vi "e.gate HighSpeedPort Decode Diagnostic Data.vi"(8 "error in":errorcluster, 10 "IsBigEndian":i32, 11 "Binary Data in":u8[](array[numeric])) -> (0 "error out":errorcluster, 1 "Error Count":i32[](array[numeric]), 2 "Cycle Count":i32[](array[numeric]), 3 "Remaining Binary Data":u8[](array[numeric]), 4 "DeltaTimeS":dbl[](array[numeric]), 5 "Error States":i16[](array[numeric]), 7 "Global Indexs":i16[](array[numeric]))   [LabVIEW 2016]
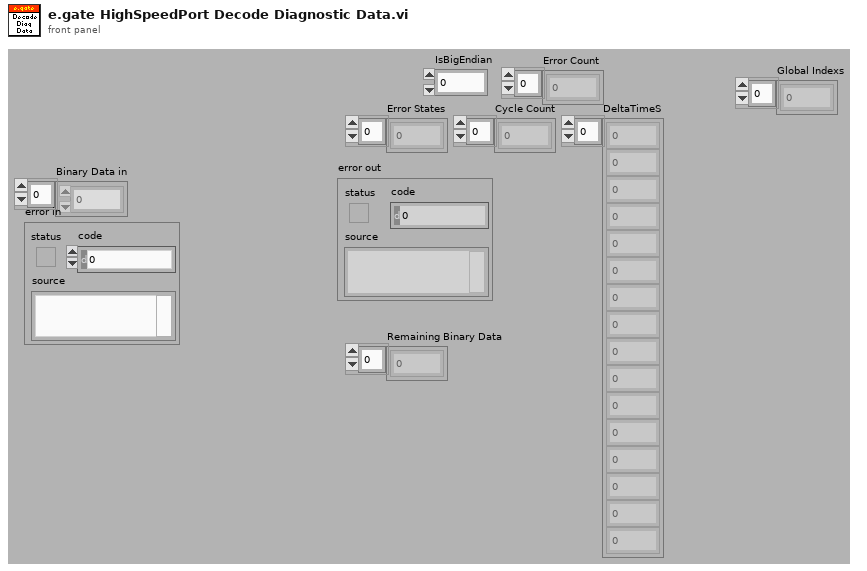
[diagram p1: front panel]
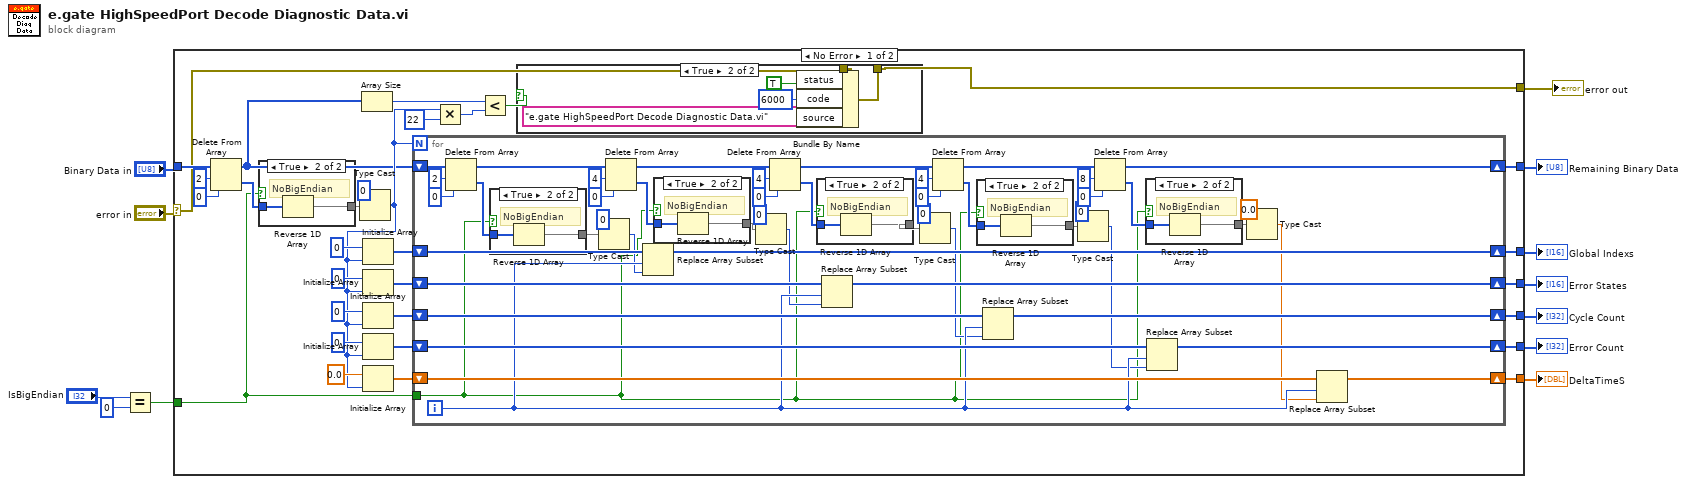
[diagram p0: block diagram]
diagram:
  n1 = Equal?(x="IsBigEndian", y=0) -> (x = y?=w1:bool)
  n2 = case shown="No Error" "error in" {
    selector: "error in" -> [w20 w116]
    tunnel: "Binary Data in" -> [w40 _]
    tunnel: [w29 _] -> w4
    tunnel: [w28 _] -> w9
    tunnel: [w27 _] -> w8
    tunnel: [w26 _] -> w7
    tunnel: [w25 _] -> w6
    tunnel: [w24 _] -> w5
    tunnel: [w16 w116] -> w10
    tunnel: w1 -> [w13 _]
    frame No Error {
      n3 = Delete From Array(array=w40, length=2 ("Länge"), index=0 ("Index")) -> (deleted portion=w15:u8[], array with subset deleted=w21:u8[])
      n4 = case shown="True" w13 {
        tunnel: w15 -> [w44 w46]
        tunnel: [w44 w45] -> w14
        frame False {
        }
        frame True {
          # "NoBigEndian"
          n5 = Reverse 1D Array(array=w46) -> (reversed array=w45:u8[])
        }
      }
      n6 = Type Cast(type=i16 0, x=w14) -> (*(type *) &x=w23:i16)
      n7 = Array Size(array=w21) -> (size(s)=w19:i32)
      n8 = Initialize Array(i16 0, w23) -> (w39:i16[])
      n9 = Initialize Array(i16 0, w23) -> (w35:i16[])
      n10 = Initialize Array(0 ("Element"), w23) -> (w34:i32[])
      n11 = Initialize Array(0 ("Element"), w23) -> (w31:i32[])
      n12 = Initialize Array(0.0 ("Element"), w23) -> (w30:dbl[])
      n13 = for {
        N: w23 -> [_]
        shift-right: [w86] -> w24
        shift-left: w21 -> [w85]
        shift-right: [w83] -> w29
        shift-left: w39 -> [w84]
        shift-right: [w81] -> w28
        shift-left: w35 -> [w82]
        shift-right: [w79] -> w27
        shift-left: w34 -> [w80]
        shift-right: [w77] -> w26
        shift-left: w31 -> [w78]
        shift-right: [w75] -> w25
        shift-left: w30 -> [w76]
        tunnel: w13 -> [w54]
        i -> [w74]
        n14 = Delete From Array(array=w85, length=2 ("Länge"), index=0 ("Index")) -> (deleted portion=w63:u8[], array with subset deleted=w96:u8[])
        n15 = case shown="True" w54 {
          tunnel: w63 -> [w113 w115]
          tunnel: [w113 w114] -> w62
          frame False {
          }
          frame True {
            # "NoBigEndian"
            n16 = Reverse 1D Array(array=w115) -> (reversed array=w114:u8[])
          }
        }
        n17 = Type Cast(type=i16 0, x=w62) -> (*(type *) &x=w64:i16)
        n18 = Delete From Array(array=w96, length=4 ("Länge"), index=0 ("Index")) -> (deleted portion=w61:u8[], array with subset deleted=w89:u8[])
        n19 = Replace Array Subset(array=w84, new element=w64, index=w74) -> (w83:i16[])
        n20 = case shown="True" w54 {
          tunnel: w61 -> [w110 w112]
          tunnel: [w110 w111] -> w60
          frame False {
          }
          frame True {
            # "NoBigEndian"
            n21 = Reverse 1D Array(array=w112) -> (reversed array=w111:u8[])
          }
        }
        n22 = Type Cast(type=0, x=w60) -> (*(type *) &x=w69:i32)
        n23 = Delete From Array(array=w89, length=4 ("Länge"), index=0 ("Index")) -> (deleted portion=w59:u8[], array with subset deleted=w88:u8[])
        n24 = case shown="True" w54 {
          tunnel: w59 -> [w107 w109]
          tunnel: [w107 w108] -> w58
          frame False {
          }
          frame True {
            # "NoBigEndian"
            n25 = Reverse 1D Array(array=w109) -> (reversed array=w108:u8[])
          }
        }
        n26 = Replace Array Subset(array=w82, new element=w69, index=w74) -> (w81:i16[])
        n27 = Type Cast(type=0, x=w58) -> (*(type *) &x=w68:i32)
        n28 = Delete From Array(array=w88, length=4 ("Länge"), index=0 ("Index")) -> (deleted portion=w57:u8[], array with subset deleted=w87:u8[])
        n29 = case shown="True" w54 {
          tunnel: w57 -> [w104 w106]
          tunnel: [w104 w105] -> w56
          frame False {
          }
          frame True {
            # "NoBigEndian"
            n30 = Reverse 1D Array(array=w106) -> (reversed array=w105:u8[])
          }
        }
        n31 = Replace Array Subset(array=w80, new element=w68, index=w74) -> (w79:i32[])
        n32 = Type Cast(type=0, x=w56) -> (*(type *) &x=w67:i32)
        n33 = Delete From Array(array=w87, length=8 ("Länge"), index=0 ("Index")) -> (deleted portion=w55:u8[], array with subset deleted=w86:u8[])
        n34 = case shown="True" w54 {
          tunnel: w55 -> [w101 w103]
          tunnel: [w101 w102] -> w53
          frame False {
          }
          frame True {
            # "NoBigEndian"
            n35 = Reverse 1D Array(array=w103) -> (reversed array=w102:u8[])
          }
        }
        n36 = Replace Array Subset(array=w78, new element=w67, index=w74) -> (w77:i32[])
        n37 = Type Cast(type=0.0, x=w53) -> (*(type *) &x=w66:dbl)
        n38 = Replace Array Subset(array=w76, new element=w66, index=w74) -> (w75:dbl[])
      }
      n39 = Multiply(x=w23, y=i16 22) -> (x*y=w18:i16)
      n40 = Less?(x=w19, y=w18) -> (x < y?=w17:bool)
      n41 = case shown="True" w17 {
        tunnel: w20 -> [w47 w52]
        tunnel: [w47 w51] -> w16
        frame False {
        }
        frame True {
          n42 = Bundle By Name(cluster=w52, "status"=TRUE, "code"=6000, "source"="e.gate HighSpeedPort Decode Diagnostic Data.vi") -> (w51:errorcluster)
        }
      }
    }
    frame Error {
    }
  }
  "error out" <- w10
  "Error States" <- w9
  "Cycle Count" <- w8
  "Error Count" <- w7
  "DeltaTimeS" <- w6
  "Remaining Binary Data" <- w5
  "Global Indexs" <- w4
